vi "Get Object by Class name new.vi"(8 "error in (no error)":errorcluster, 10 "Class Name":string, 11 "Cache Manager DVR in":refnum<class "Cache Manager.lvclass">) -> (0 "error out":errorcluster, 2 "Serializable Message":refnum<class "Serializable Msg.lvclass">, 3 "Cache Manager DVR out":refnum<class "Cache Manager.lvclass">)   [LabVIEW 2020, in "Cache Manager.lvclass"]
uses:
  Cache Manager.lvclass
  Serializer/Serializable Message/Serializable Msg.lvclass
  Cache Manager.lvclass/Cache Manager.ctl
  <vilib>/Utility/miscctls.llb/LVMapReplaceAction.ctl
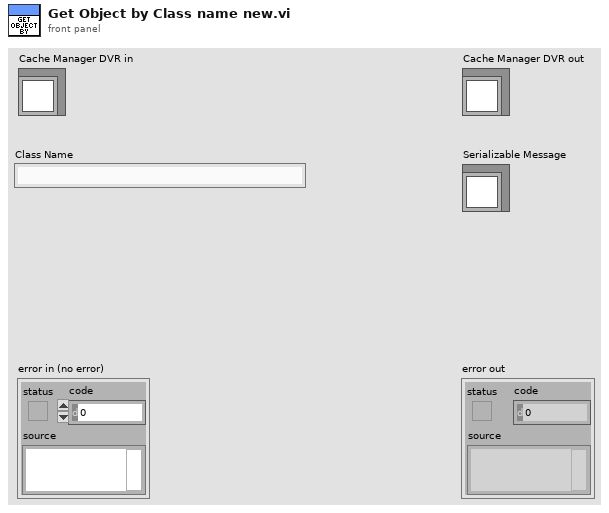
[diagram p1: front panel]
types:
  T1 = typedef "LVMapReplaceAction.ctl" = enum32{"Modify Entry only if found", "Add or Modify Entry", "Delete Entry"}
  T2 = map{string, refnum<class "Serializable Msg.lvclass">}
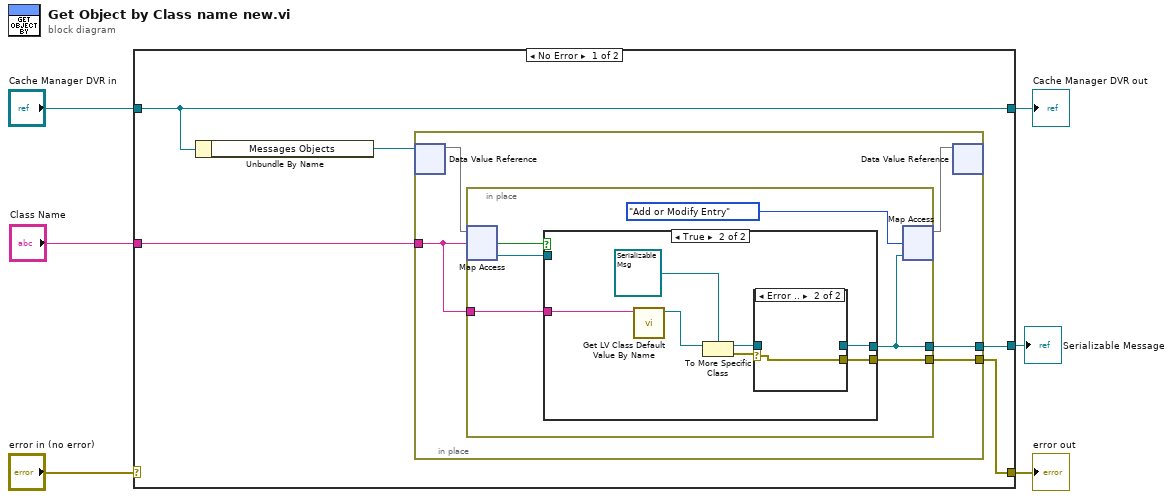
[diagram p0: block diagram]
diagram:
  n1 = case shown="No Error" "error in (no error)" {
    selector: "error in (no error)" -> [_ w34]
    tunnel: [w7 w34] -> w5
    tunnel: [w11 w33] -> w3
    tunnel: "Cache Manager DVR in" -> [w11 w33]
    tunnel: "Class Name" -> [w9 _]
    tunnel: [w8 _] -> w1
    frame No Error {
      n2 = Unbundle By Name(w11) -> ("Messages Objects"=w10:refnum<data-value>)
      n3 = in-place "In Place Element Structure" {
        in-place-border: w9 -> [w14]
        in-place-border: [w15] -> w8
        in-place-border: [w12] -> w7
        n4 = in-place-dvr #1(w10) -> (w16:T2)  [unwired: 1 out]
        n5 = in-place "In Place Element Structure" {
          in-place-border: [w18] -> w15
          in-place-border: w14 -> [w19]
          in-place-border: [w17] -> w12
          n6 = in-place-map #2(w16, w14) -> (w20:refnum<class "Serializable Msg.lvclass">, w21:bool)  [unwired: 1 in]
          n7 = case shown="True" w21 {
            tunnel: w20 -> [w23 _]
            tunnel: [w23 w25] -> w18
            tunnel: w19 -> [_ w30]
            tunnel: [_ w24] -> w17
            frame False {
            }
            frame True {
              n8 = call <vilib>:"Get LV Class Default Value By Name.vi"("class name"=w30) -> ("object"=w28:refnum<class>)  [unwired: 9 in, 1 out]
              n9 = To More Specific Class(target class=refnum<class "Serializable Msg.lvclass"> refnum ("Serializable Message.lvclass"), reference=w28) -> (specific class reference=w26:refnum<class "Serializable Msg.lvclass">, error out=w27:errorcluster)  [unwired: 1 in]
              n10 = case shown="Error .." w27 {
                selector: w27 -> [_ w32]
                tunnel: w26 -> [w31 _]
                tunnel: [w31 _] -> w25
                tunnel: [_ w32] -> w24
                frame No Error {
                }
                frame Error {
                }
              }
            }
          }
          n11 = in-place-map #2(w18, LVMapReplaceAction."Add or Modify Entry" ("action")) -> (w13:T2)  [unwired: 2 out]
        }
        n12 = in-place-dvr #1(w13) -> ()  [unwired: 2 out]
      }
    }
    frame Error {
    }
  }
  "error out" <- w5
  "Cache Manager DVR out" <- w3
  "Serializable Message" <- w1
